vi "Write Default Core.vi"(8 "error in (no error)":errorcluster, 9 "Name":string, 10 "Path":path, 11 "Cluster In":variant) -> (0 "error out":errorcluster, 3 "Cluster Out":variant)   [LabVIEW 2019, in "ObjectSettings.lvclass"]
uses:
  ObjectSettings.lvclass
  <userlib>/LevyLab/Configuration/Configuration.lvclass
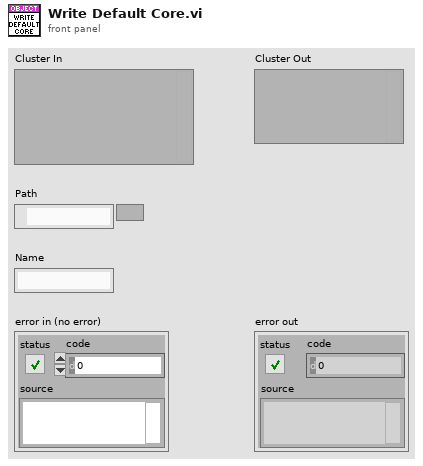
[diagram p1: front panel]
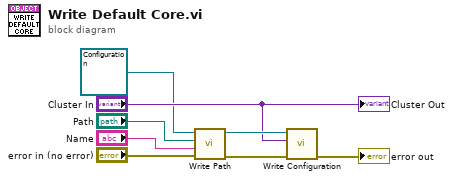
[diagram p0: block diagram]
diagram:
  n1 = call <userlib>:"Write Path.vi"("error in (no error)"="error in (no error)", "Filename [Configuration.ini]"="Name", "Path"="Path", "Configuration in"=refnum<class "Configuration.lvclass"> refnum) -> ("error out"=w7:errorcluster, "Configuration out"=w8:refnum<class "Configuration.lvclass">)  [unwired: 6 in]
  n2 = call <userlib>:"Write Configuration.vi"("error in (no error)"=w7, "Variant"="Cluster In", "Configuration in"=w8) -> ("error out"=→"error out":errorcluster)  [unwired: 7 in, 1 out]
  "Cluster Out" <- "Cluster In"
